vi "testDataPass_v1,0_vi1.vi"() -> ()   [LabVIEW 2014]
panel:
  out "error out":errorcluster
  in  "stop":bool
  in  "arrTF_write":bool[](array[boolean])
  in  "Write Location":string="dstp://localhost/wave"
  # "Run the DataSocket server by navigating the Windows start menu to National Instruments > DataSocket > DataSocket Server."
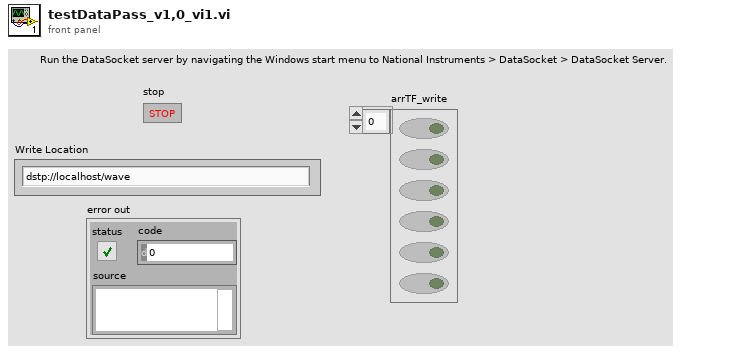
[diagram p1: front panel]
types:
  T1 = enum16{"Read", "Write", "ReadWrite", "BufferedRead", "BufferedReadWrite"}
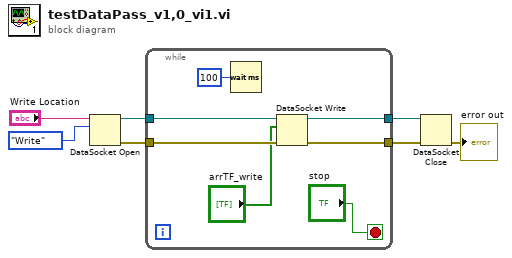
[diagram p0: block diagram]
diagram:
  n1 = DataSocket Open(10:T1."Write" ("mode"), 11:"Write Location") -> (0:w4:errorcluster, 3:w5:refnum<k13>)  [unwired: 2 in]
  n2 = while {
    tunnel: w5 -> [w13]
    tunnel: w4 -> [w12]
    tunnel: [w9] -> w3
    tunnel: [w8] -> w2
    stop <- "stop" stop-if-true
    n3 = Wait (ms)(milliseconds to wait=u32 100) -> ()  [unwired: 1 out]
    n4 = DataSocket Write(8:w12, 10:"arrTF_write", 11:w13) -> (0:w8:errorcluster, 3:w9:refnum<k13>)  [unwired: 2 out]
  }
  n5 = DataSocket Close(8:w2, 11:w3) -> (0:→"error out":errorcluster)  [unwired: 1 in, 1 out]
